vi "etc_XCITE_OpenDevice.vi"(0 "h":u64, 1 "type":i32(ring)=65535 items=["XC_120PC"=0, "XC_exacte"=1, "XC_120LED"=2, "XC_110LED"=3, "XC_mini"=4, "XC_XYLIS"=5, "XC_XR210"=6, "XC_LED1"=7, "XC_XT600"=8, "XC_XT900"=9, "Any"=65535], 2 "port":string, 3 "baudrate":u32=9600, 5 "error in (no error)":errorcluster {"code" format="%x"}) -> (14 "h out":u64, 15 "ErrorMessage":i32 format="%x", 19 "error out":errorcluster {"code" format="%x"})   [LabVIEW 2019, in "XCite.lvlib"]
doc: "Opens communication with the slelected X-cite device."
uses:
  XCite.lvlib
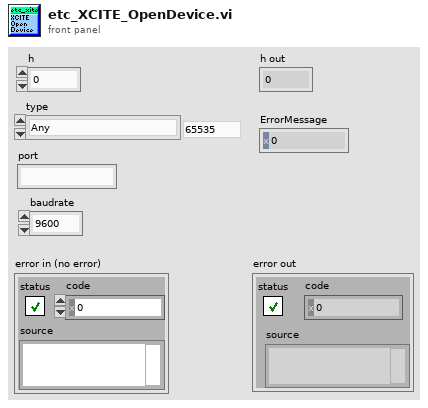
[diagram p1: front panel]
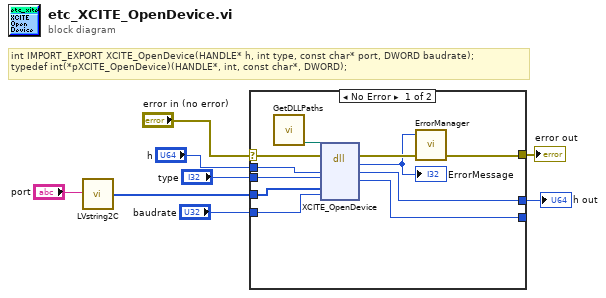
[diagram p0: block diagram]
diagram:
  # "int IMPORT_EXPORT XCITE_OpenDevice(HANDLE* h, int type, const char* port, DWORD baudrate);\ntypedef int(*pXCITE_OpenDevice)(HANDLE*, int, const char*, DWORD);"
  n1 = call "LVstring2C.vi"("LVString"="port") -> ("CString"=w2:u8[])  [unwired: 3 in, 1 out]
  n2 = case shown="No Error" "error in (no error)" {
    selector: "error in (no error)" -> [w19 w22]
    tunnel: [w17 w22] -> w8
    tunnel: "h" -> [w15 w21]
    tunnel: [w14 w21] -> w6
    tunnel: "baudrate" -> [w12 _]
    tunnel: "type" -> [w11 w20]
    tunnel: [w10 w20] -> _
    tunnel: w2 -> [w9 _]
    frame No Error {
      n3 = call "GetDLLPaths.vi"() -> ("etc_xcite_path"=w13:path)  [unwired: 8 in, 3 out]
      n4 = dll-call lib="C:/LabVIEWDevFall2024/pco.labview/labview_sdk/runtime/bin64/etc_xcite.dll" fn="XCITE_OpenDevice"(path in=w13, error in=w19, "h"=w15, "type"=w11, "port"=w9, "baudrate"=w12) -> (error out=w18:errorcluster, "return type"=w16:i32, "h"=w14:u64, "type"=w10:i32)  [unwired: 3 in, 1 out]
      "ErrorMessage" <- w16
      n5 = call "ErrorManager.vi"("error in (no error)"=w18, "error code"=w16) -> ("error out"=w17:errorcluster)  [unwired: 2 in, 1 out]
    }
    frame Error {
    }
  }
  "error out" <- w8
  "h out" <- w6
